vi "Teleop.vi"(10 "Match Info":T1={"Autonomous Elapsed Seconds"=0.0, "TeleOp Elapsed Seconds"=0.0, "Disabled Elapsed Seconds"=0.0, "Visited Autonomous"=FALSE, "Visited TeleOp"=FALSE, "Visited Disabled"=FALSE, "Autonomous Settings"={"Autonomous Style"=enum."Independent", "VI Refnum"=refnum}}, 11 "Call Context":T2) -> ()   [LabVIEW 2015]
doc: "This VI is called for each TeleOp packet received from the DS where the robot is not disabled. It is often used to read from the joysticks and update I/O or to update setpoints for timed control loops. It should complete and return within 20 milliseconds or it may miss DS packets."
uses:
  <vilib>/Rock Robotics/WPI/DriverStation/WPI_DriverStationDerivedRobotMode.ctl
  <vilib>/Rock Robotics/WPI/DriverStation/WPI_DriverStationMatch Info.ctl
  <vilib>/Rock Robotics/WPI/Solenoid/WPI_SolenoidValue.ctl
  <vilib>/Rock Robotics/Network Tables/NT Read Boolean.vi
  <vilib>/Rock Robotics/Network Tables/NT Read Number.vi
  <vilib>/Rock Robotics/WPI/Utilities/WPI_GetSetVariantRefNum.vi
  <vilib>/Rock Robotics/WPI/Solenoid/WPI_SolenoidSetEnum.vi
panel:
  in  "Numeric":dbl
  out "Encodeur gauche min":dbl
  out "Encodeur gauche max":dbl
  out "Encodeur droit max":dbl
  out "Encodeur droit min":dbl
  out "Sample Slider 0":dbl(slide) scale=0.0..5.0
  out "Sample Boolean 1":bool
  out "Sample Boolean 0":bool
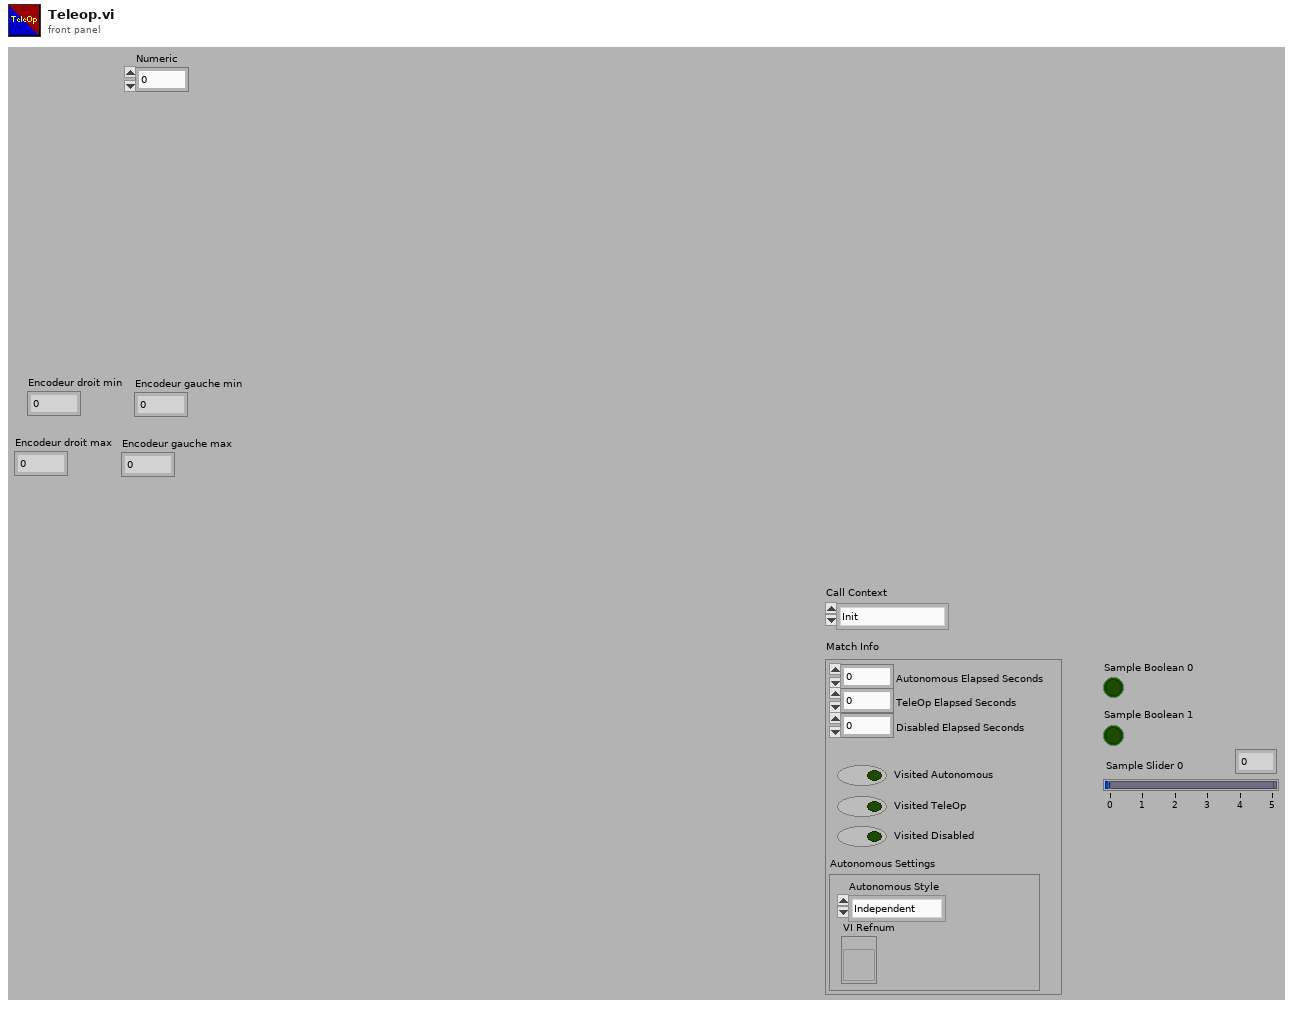
[diagram p1: front panel]
types:
  T1 = typedef "WPI_DriverStationMatch Info.ctl" = cluster{"Autonomous Elapsed Seconds":dbl, "TeleOp Elapsed Seconds":dbl, "Disabled Elapsed Seconds":dbl, "Visited Autonomous":bool, "Visited TeleOp":bool, "Visited Disabled":bool, "Autonomous Settings":cluster{"Autonomous Style":enum16{"Iterative", "Independent"}, "VI Refnum":refnum<vi>}}
  T2 = typedef "WPI_DriverStationDerivedRobotMode.ctl" = enum16{"Init", "Execute", "Stop"}
  T3 = typedef "WPI_JoystickDevRef.ctl" = cluster{"Device":T4}
  T4 = typedef "WPI_JoystickDeviceEnum.ctl" = enum16{"USB 0", "USB 1", "USB 2", "USB 3", "USB 4", "USB 5"}
  T5 = typedef "WPI_EncoderDevRef.ctl" = cluster{"DevStatus":errorcluster, "EncoderIndex":T6, "CounterIndex":T7, "DistancePerCount":dbl, "Decoding Type":T8}
  T6 = typedef "FPGA_EncoderIdx.ctl" = enum8{"Enc 0", "Enc 1", "Enc 2", "Enc 3", "Enc 4", "Enc 5", "Enc 6", "Enc 7", "Invalid"}
  T7 = typedef "FPGA_CounterCtrSystemIndex.ctl" = enum8{"Ctr 0", "Ctr 1", "Ctr 2", "Ctr 3", "Ctr 4", "Ctr 5", "Ctr 6", "Ctr 7", "Invalid"}
  T8 = typedef "WPI_EncoderType.ctl" = enum16{"1x", "2x", "4x"}
  T9 = cluster{"Axes[0]":dbl, "Axes[1]":dbl, "Axes[2]":dbl, "Axes[3]":dbl, "Axes[4]":dbl, "Axes[5]":dbl, "Axes[6]":dbl, "Axes[7]":dbl, "Axes[8]":dbl}
  T10 = cluster{"Buttons[0]":bool, "Buttons[1]":bool, "Buttons[2]":bool, "Buttons[3]":bool, "Buttons[4]":bool, "Buttons[5]":bool, "Buttons[6]":bool, "Buttons[7]":bool, "Buttons[8]":bool}
  T11 = typedef "WPI_MotorControlDeviceRef.ctl" = cluster{"DeviceStatus":errorcluster, "Type":T12, "PWM":cluster{"PWM Channel":T13, "DeadBand":T14}, "CAN":cluster{"Device Number":u8, "Control Mode":T15, "Semaphore":T16, "Max Vout":dbl, "TalonSRX Control Mode":T17}, "Invert":bool}
  T12 = typedef "WPI_MotorControlType.ctl" = enum16{"PWM", "CAN", "CANTalonSRX"}
  T13 = typedef "FPGA_DIOPWMChannel.ctl" = enum8{"PWM 0", "PWM 1", "PWM 2", "PWM 3", "PWM 4", "PWM 5", "PWM 6", "PWM 7", "PWM 8", "PWM 9", "PWM MXP 0", "PWM MXP 1", "PWM MXP 2", "PWM MXP 3", "PWM MXP 4", "PWM MXP 5", "PWM MXP 6", "PWM MXP 7", "PWM MXP 8", "PWM MXP 9", "Invalid"}
  T14 = typedef "WPI_PWMDeadband.ctl" = cluster{"Name":string, "maxPositivePwm":i32, "minPositivePwm":i32, "centerPwm":i32, "maxNegativePwm":i32, "minNegativePwm":i32, "angularRange":u16}
  T15 = typedef "WPI_CANJaguar_ControlMode.ctl" = enum8{"Percent VBus", "Current", "Speed", "Position", "Voltage"}
  T16 = typedef "Semaphore RefNum" = refnum<k1>
  T17 = typedef "WPI_CANTalonSRX_APIControlMode.ctl" = enum8{"Percent VBus", "Speed", "Position", "Slave", "Unchanged / Invalid", "Voltage Compensation", "Current", "Motion Profile"}
  T18 = typedef "WPI_SolenoidDevRef.ctl" = cluster{"DevStatus":errorcluster, "Pneumatics Control Module":u8, "Forward Solenoid Channel":T19, "Reverse Solenoid Channel":T19}
  T19 = typedef "WPI_SolenoidChannel.ctl" = enum8{"Solenoid 0", "Solenoid 1", "Solenoid 2", "Solenoid 3", "Solenoid 4", "Solenoid 5", "Solenoid 6", "Solenoid 7", "Invalid"}
  T20 = typedef "WPI_SolenoidValue.ctl" = enum16{"Off", "On", "Forward", "Reverse"}
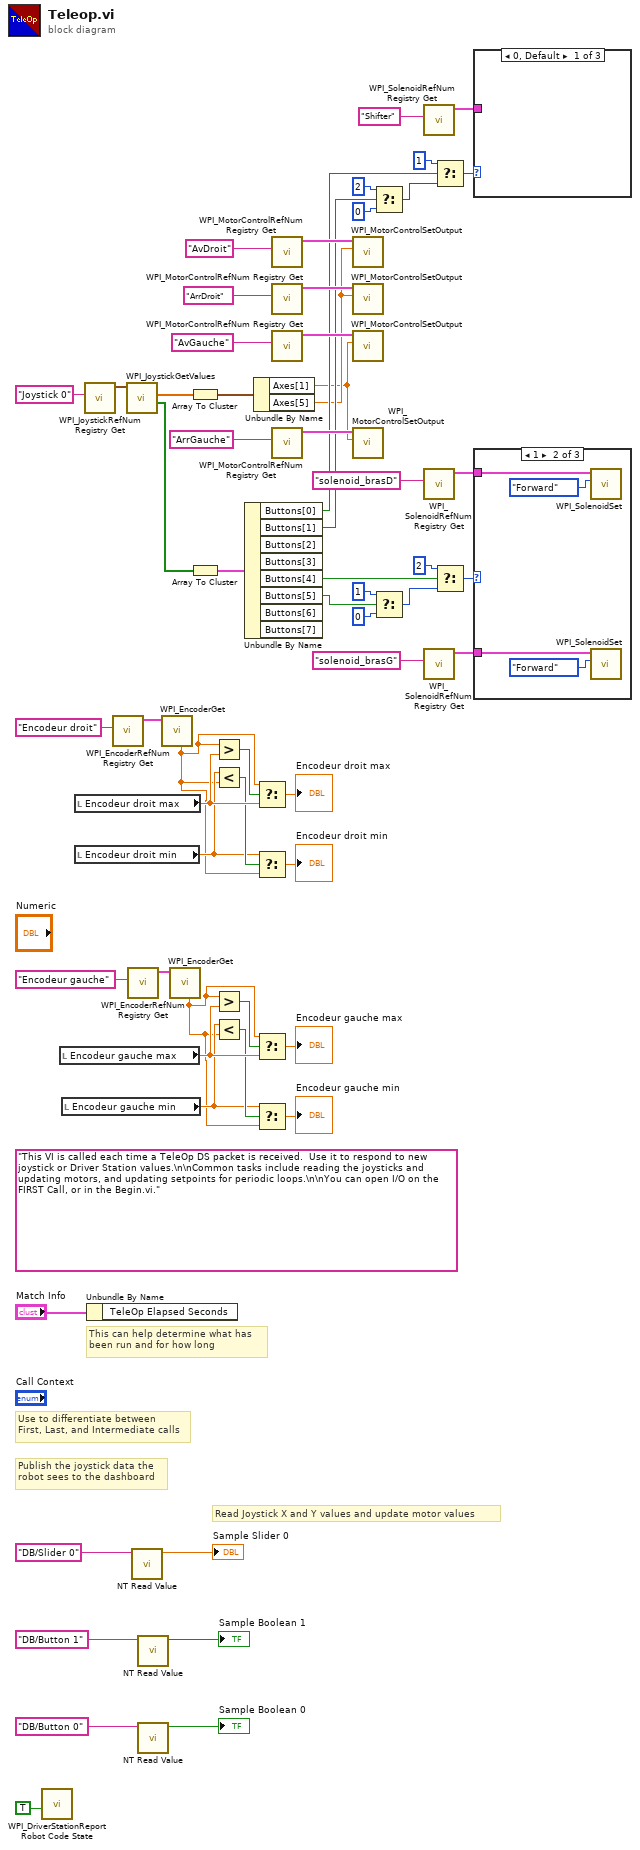
[diagram p0: block diagram]
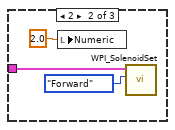
[diagram p2: hidden frame]
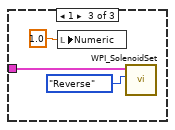
[diagram p3: hidden frame]
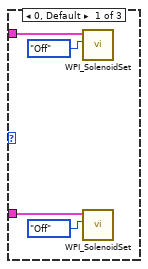
[diagram p4: hidden frame]
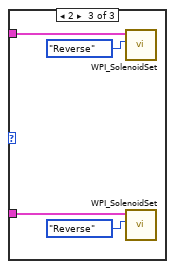
[diagram p5: hidden frame]
diagram:
  (unwired) "This VI is called each time a TeleOp DS packet is received.  Use it to respond to new joystick or Driver Station values.\n\nCommon tasks include reading the joysticks and updating motors, and updating setpoints for periodic loops.\n\nYou can open I/O on the FIRST Call, or in the Begin.vi."
  # "Publish the joystick data the\nrobot sees to the dashboard"
  # "Use to differentiate between\nFirst, Last, and Intermediate calls"
  # "This can help determine what has\nbeen run and for how long"
  # "Read Joystick X and Y values and update motor values"
  n1 = call <vilib>:"WPI_DriverStationReport Robot Code State.vi"("TeleOp"=TRUE ("Autonomous")) -> ()  [unwired: 10 in, 1 out]
  n2 = local read "Encodeur gauche max"() -> (w34:dbl)
  n3 = local read "Encodeur gauche min"() -> (w31:dbl)
  n4 = local read "Encodeur droit max"() -> (w29:dbl)
  n5 = local read "Encodeur droit min"() -> (w27:dbl)
  n6 = call <vilib>:"WPI_JoystickRefNum Registry Get.vi"("refnum name"="Joystick 0") -> ("JoystickDevRef"=w53:T3)  [unwired: 1 in, 9 out]
  n7 = Unbundle By Name("Match Info") -> ()  [unwired: 1 out]
  n8 = call <vilib>:"WPI_EncoderRefNum Registry Get.vi"("refnum name"="Encodeur droit") -> ("EncoderDevRef"=w38:T5)  [unwired: 9 in, 1 out]
  n9 = call <vilib>:"WPI_JoystickGetValues.vi"("JoystickDevRef"=w53) -> ("Buttons"=w50:bool[], "Axes"=w52:dbl[])  [unwired: 6 in, 3 out]
  n10 = call <vilib>:"WPI_EncoderRefNum Registry Get.vi"("refnum name"="Encodeur gauche") -> ("EncoderDevRef"=w37:T5)  [unwired: 9 in, 1 out]
  n11 = call-poly <vilib>:"NT Read Value.vi"("Name"="DB/Slider 0" ("refnum name")) -> ("Numeric"=→"Sample Slider 0":dbl)  [unwired: 9 in, 1 out]
  n12 = call-poly <vilib>:"NT Read Value.vi"("Name"="DB/Button 1" ("refnum name")) -> ("Boolean"=→"Sample Boolean 1":bool)  [unwired: 9 in, 1 out]
  n13 = call-poly <vilib>:"NT Read Value.vi"("Name"="DB/Button 0" ("refnum name")) -> ("Boolean"=→"Sample Boolean 0":bool)  [unwired: 9 in, 1 out]
  n14 = call <vilib>:"WPI_EncoderGet.vi"("EncoderDevRef"=w38) -> ("Rate"=w3:dbl)  [unwired: 5 in, 5 out]
  n15 = call <vilib>:"WPI_EncoderGet.vi"("EncoderDevRef"=w37) -> ("Rate"=w16:dbl)  [unwired: 5 in, 5 out]
  n16 = Array To Cluster(array=w52) -> (cluster=w51:T9)
  n17 = Array To Cluster(array=w50) -> (cluster=w8:T10)
  n18 = Greater?(x=w3, y=w29) -> (0:w30:bool)
  n19 = Less?(x=w27, y=w3) -> (x < y?=w28:bool)
  n20 = Greater?(x=w16, y=w34) -> (0:w35:bool)
  n21 = Less?(x=w31, y=w16) -> (x < y?=w32:bool)
  n22 = Unbundle By Name(w8) -> ("Buttons[0]"=w7:bool, "Buttons[1]"=w6:bool, "Buttons[4]"=w5:bool, "Buttons[5]"=w4:bool)  [unwired: 4 out]
  n23 = Unbundle By Name(w51) -> ("Axes[1]"=w1:dbl, "Axes[5]"=w2:dbl)
  n24 = Select(t=w3, s=w30, f=w29) -> (s? t:f=→"Encodeur droit max":dbl)
  n25 = Select(t=w27, s=w28, f=w3) -> (s? t:f=→"Encodeur droit min":dbl)
  n26 = Select(t=w16, s=w35, f=w34) -> (s? t:f=→"Encodeur gauche max":dbl)
  n27 = Select(t=w31, s=w32, f=w16) -> (s? t:f=→"Encodeur gauche min":dbl)
  n28 = call <vilib>:"WPI_MotorControlRefNum Registry Get.vi"("refnum name"="AvDroit") -> ("MotorControlDevRef"=w22:T11)  [unwired: 9 in, 1 out]
  n29 = call <vilib>:"WPI_MotorControlRefNum Registry Get.vi"("refnum name"="ArrDroit") -> ("MotorControlDevRef"=w21:T11)  [unwired: 9 in, 1 out]
  n30 = call <vilib>:"WPI_MotorControlRefNum Registry Get.vi"("refnum name"="AvGauche") -> ("MotorControlDevRef"=w24:T11)  [unwired: 9 in, 1 out]
  n31 = call <vilib>:"WPI_MotorControlRefNum Registry Get.vi"("refnum name"="ArrGauche") -> ("MotorControlDevRef"=w23:T11)  [unwired: 9 in, 1 out]
  n32 = call <vilib>:"WPI_MotorControlSetOutput.vi"("Output"=w2, "MotorControlDevRef"=w22) -> ()  [unwired: 7 in, 3 out]
  n33 = call <vilib>:"WPI_MotorControlSetOutput.vi"("Output"=w2, "MotorControlDevRef"=w21) -> ()  [unwired: 7 in, 3 out]
  n34 = call <vilib>:"WPI_MotorControlSetOutput.vi"("Output"=w1, "MotorControlDevRef"=w24) -> ()  [unwired: 7 in, 3 out]
  n35 = call <vilib>:"WPI_MotorControlSetOutput.vi"("Output"=w1, "MotorControlDevRef"=w23) -> ()  [unwired: 7 in, 3 out]
  n36 = Select(t=2, s=w6, f=0) -> (s? t:f=w47:i32)
  n37 = Select(t=1, s=w4, f=0) -> (s? t:f=w45:i32)
  n38 = call <vilib>:"WPI_SolenoidRefNum Registry Get.vi"("refnum name"="Shifter") -> ("SolenoidDevRef"=w14:T18)  [unwired: 9 in, 1 out]
  n39 = call <vilib>:"WPI_SolenoidRefNum Registry Get.vi"("refnum name"="solenoid_brasD") -> ("SolenoidDevRef"=w9:T18)  [unwired: 9 in, 1 out]
  n40 = call <vilib>:"WPI_SolenoidRefNum Registry Get.vi"("refnum name"="solenoid_brasG") -> ("SolenoidDevRef"=w40:T18)  [unwired: 9 in, 1 out]
  n41 = Select(t=1, s=w7, f=w47) -> (s? t:f=w13:i32)
  n42 = Select(t=2, s=w5, f=w45) -> (s? t:f=w41:i32)
  n43 = case shown="0, Default" w13 {
    tunnel: w14 -> [_ w65 w67]
    frame 0, Default {
    }
    frame 2 {
      n44 = local write "Numeric"(2.0 ("Numeric")) -> ()
      n45 = call-poly <vilib>:"WPI_SolenoidSet.vi"("Value"=WPI_SolenoidValue."Forward", "SolenoidDevRef"=w65) -> ()  [unwired: 8 in, 2 out]
    }
    frame 1 {
      n46 = local write "Numeric"(1.0 ("Numeric")) -> ()
      n47 = call-poly <vilib>:"WPI_SolenoidSet.vi"("Value"=WPI_SolenoidValue."Reverse", "SolenoidDevRef"=w67) -> ()  [unwired: 8 in, 2 out]
    }
  }
  n48 = case shown="1" w41 {
    tunnel: w40 -> [w71 w76 w79]
    tunnel: w9 -> [w69 w73 w77]
    frame 0, Default {
      n49 = call-poly <vilib>:"WPI_SolenoidSet.vi"("Value"=WPI_SolenoidValue."Off", "SolenoidDevRef"=w69) -> ()  [unwired: 8 in, 2 out]
      n50 = call-poly <vilib>:"WPI_SolenoidSet.vi"("Value"=WPI_SolenoidValue."Off", "SolenoidDevRef"=w71) -> ()  [unwired: 8 in, 2 out]
    }
    frame 1 {
      n51 = call-poly <vilib>:"WPI_SolenoidSet.vi"("Value"=WPI_SolenoidValue."Forward", "SolenoidDevRef"=w73) -> ()  [unwired: 8 in, 2 out]
      n52 = call-poly <vilib>:"WPI_SolenoidSet.vi"("Value"=WPI_SolenoidValue."Forward", "SolenoidDevRef"=w76) -> ()  [unwired: 8 in, 2 out]
    }
    frame 2 {
      n53 = call-poly <vilib>:"WPI_SolenoidSet.vi"("Value"=WPI_SolenoidValue."Reverse", "SolenoidDevRef"=w77) -> ()  [unwired: 8 in, 2 out]
      n54 = call-poly <vilib>:"WPI_SolenoidSet.vi"("Value"=WPI_SolenoidValue."Reverse", "SolenoidDevRef"=w79) -> ()  [unwired: 8 in, 2 out]
    }
  }
